vi "Anisotropic Filter Example.vi"() -> ()   [LabVIEW 2012]
uses:
  Non-User VIs/Controls/Anisotropic Filter Parameters.ctl
  User Controls/Array Dimensions.ctl
  <vilib>/Analysis/baseanly.llb/Scale 2D.vi
  Non-User VIs/Allocate Memory/AllocateMemory_32f.vi
  Non-User VIs/Functions/Anisotropic Filter/Create Ansiotropic Filter 32f.vi
  Non-User VIs/Functions/Anisotropic Filter/Compute Anisotropic Filter 32f.vi
  Non-User VIs/Functions/Anisotropic Filter/Delete Ansiotropic Filter 32f.vi
  Non-User VIs/Error Checking/View Error Log Mode Functional Global.vi
  OpenCLV x64.lvlib
  <vilib>/Analysis/NI_AALBase.lvlib
panel:
  in  "Ansiotropic Filter Parameters":T1={"Time Step"=0.1, "Total Time"=0.5, "Std. Deviation"=1.6, "Gaussian Filter X Size"=3, "Gaussian Filter Y Size"=3, "Gaussian Filter Z Size"=3} {"Gaussian Filter Z Size" min=1 max=99 step=2; "Gaussian Filter Y Size" min=1 max=99 step=2; "Gaussian Filter X Size" min=1 max=99 step=2}
  out "Normalized Raw Image":dbl[][](graph)
  out "Normalized Proessed Image":dbl[][](graph)
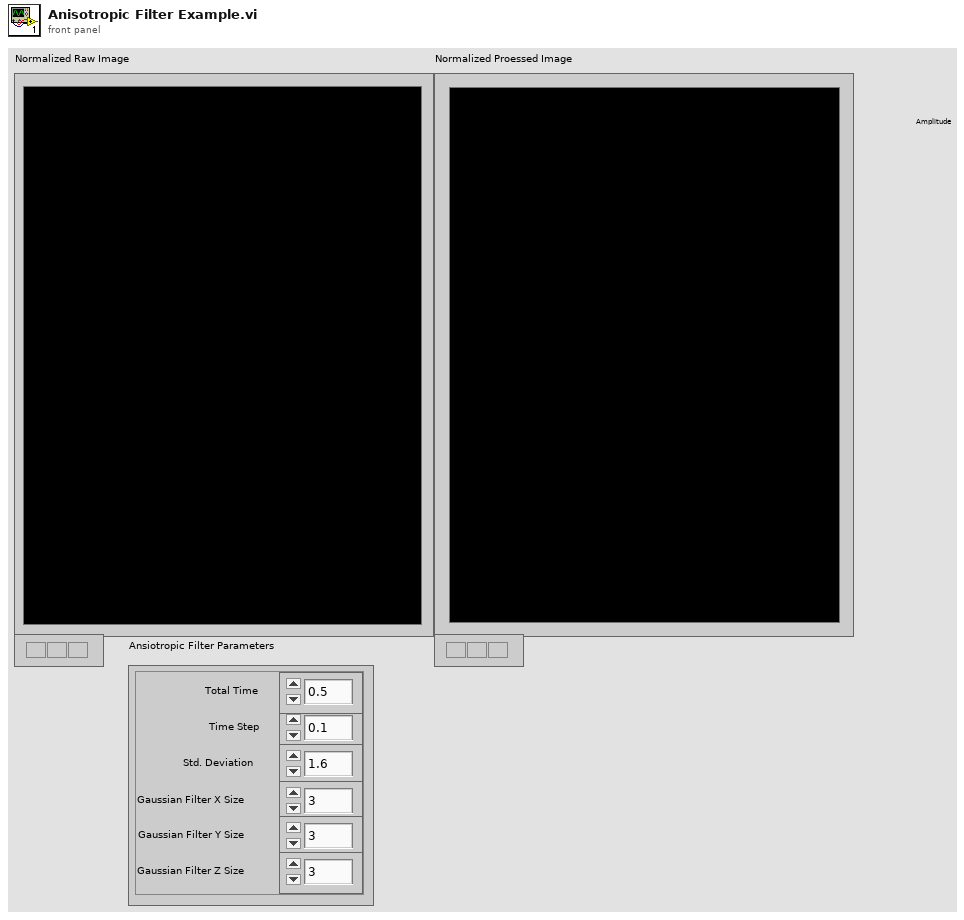
[diagram p1: front panel]
types:
  T1 = typedef "OpenCLV x64.lvlib/Anisotropic Filter Parameters.ctl" = cluster{"Time Step":sgl, "Total Time":sgl, "Std. Deviation":sgl, "Gaussian Filter X Size":u32, "Gaussian Filter Y Size":u32, "Gaussian Filter Z Size":u32}
  T2 = typedef "Array Dimensions.ctl" = cluster{"Depth":u64, "Height":u64, "Width":u64}
  T3 = typedef "imagedata.ctl" = cluster{"image type":i32, "image depth":i32, "image":u8[], "mask":u8[], "colors":u32[], "Rectangle":cluster{"left":i16, "top":i16, "right":i16, "bottom":i16}}
  T4 = typedef "OpenCLV x64.lvlib/Device ID.ctl" = u64
  T5 = typedef "OpenCLV x64.lvlib/Memory Object.ctl" = cluster{"Device ID":T4, "Memeroy ID":T6, "Dimension":T2, "Memory Type":T7}
  T6 = typedef "OpenCLV x64.lvlib/Memory ID.ctl" = u64
  T7 = typedef "OpenCLV x64.lvlib/Memory Type.ctl" = enum16{"32f", "u8", "i8", "u16", "i16", "u32", "i32", "64f"}
  T8 = typedef "OpenCLV x64.lvlib/Anisotropic Filter Object.ctl" = cluster{"Device In":T4, "Convolution Object":T9, "Imag Kernel":sgl[][][], "Real Kernel":sgl[][][], "Convolved Buffer":T5, "Program Handle":T10, "Ansiotropic Filter Parameters":T1, "Raw Data":T5, "Buffer 3":T5, "Dimensions":T2}
  T9 = typedef "OpenCLV x64.lvlib/Convolution Object.ctl" = cluster{"Device In":T4, "Program Handle":T10, "Kernel Memory Object":T5, "Convolved Memory Object":T5}
  T10 = typedef "OpenCLV x64.lvlib/Program Handle.ctl" = u64
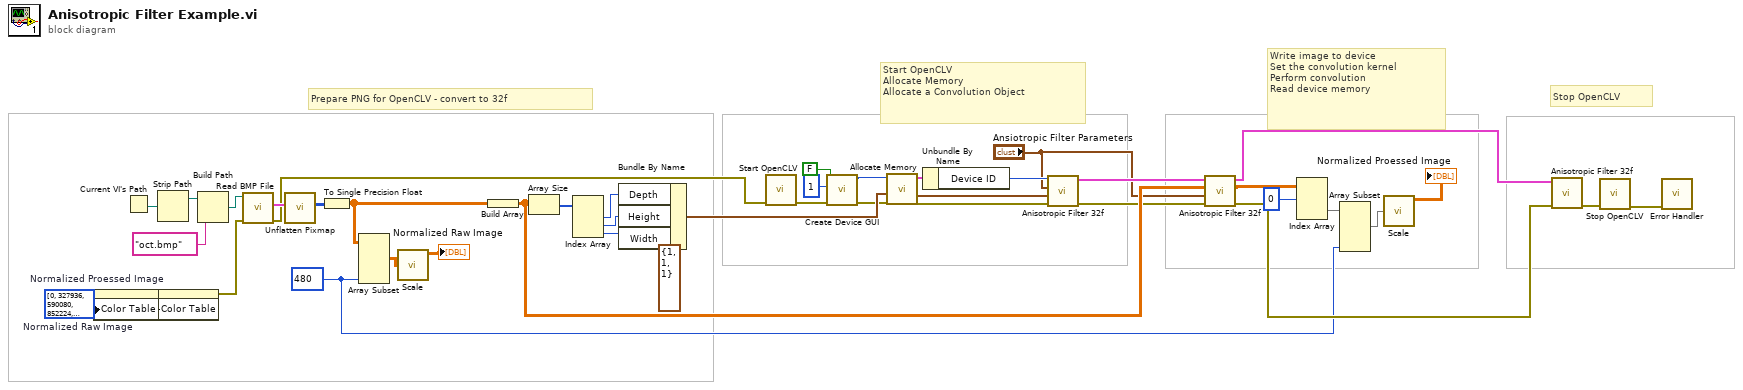
[diagram p0: block diagram]
diagram:
  w1 = 480 ("index")
  w8 = u32[] [0, 327936, 590080, 852224, 983296, 1114624, 1180160, 1311232, 1442304, 1573632, 1704704, 1770240, 1901312, 1966848, 2098176, 2163712, 2294784, 2491392, 2557184, 2688256, 2753792, 2884864, 2950656, 3081728, 3147264, 3344129, 3475457, 3540993, 3672321, 3738113, 3869185, 3934977, 4066305, 4197633, 4328961, 4394497, 4460289, 4591617, 4657409, 4788481, 4854273, 4985601, 5116929, 5248257, 5314049, 5379841, 5511169, 5576961, 5708033, 5773825, 5905153, 6036482, 6167810, 6233346, 6299138, 6430466, 6496258, 6562050, 6693634, 6759426, 6890754, 7022082, 7087874, 7153666, 7284994, 7350786, 7482114, 7547906, 7613698, 7745026, 7876354, 8007682, 8073474, 8139522, 8205314, 8336642, 8467970, 8533763, 8599555, 8665347, 8731139, 8862467, 8993795, 9059587, 9125380, 9191428, 9257220, 9388548, 9454340, 9520132, 9585924, 9717253, 9848837, 9914629, 9980165, 10045957, 10177541, 10243334, 10309126, 10375174, 10440966, 10572294, 10703623, 10769416, 10835208, 10901256, 10967049, 11033097, 11033609, 11099401, 11165450, 11231242, 11231754, 11297547, 11363339, 11429131, 11495180, 11495692, 11561740, 11693069, 11758861, 11759373, 11825165, 11891214, 11957006, 12022799, 12023311, 12089103, 12220944, 12286736, 12286736, 12352529, 12418577, 12484370, 12550162, 12615954, 12681747, 12747796, 12813588, 12813845, 12879894, 12945686, 13077015, 13142808, 13143064, 13208856, 13274905, 13340697, 13340953, 13472282, 13538075, 13604379, 13670172, 13735964, 13801757, 13867550, 13933343, 13999392, 13999648, 14065441, 14131234, 14197027, 14197541, 14263334, 14329383, 14395176, 14460969, 14592553, 14658346, 14724139, 14789932, 14790189, 14856238, 14922287, 14988080, 15053873, 15054130, 15119923, 15185972, 15251765, 15317559, 15383353, 15449146, 15449660, 15515454, 15515968, 15516226, 15582021, 15582278, 15582536, 15648587, 15648844, 15714639, 15714897, 15715155, 15780949, 15781463, 15847256, 15847770, 15848028, 15913823, 15914081, 15979875, 15980133, 15980391, 16046441, 16046444, 16046703, 16046705, 16112500, 16113015, 16113274, 16113277, 16179072, 16179330, 16179588, 16245384, 16245387, 16245389, 16245648, 16311443, 16376982, 16377241, 16377499, 16443294, 16443553, 16443555, 16443815, 16509866, 16510124, 16510127, 16575923, 16575924, 16576182, 16576441, 16576443, 16576702, 16576705, 16576963, 16577222, 16577224, 16577482, 16577485, 16577743, 16577745, 16578004, 16578262, 16578264, 16578523, 16578782, 16579040, 16579299, 16579301, 16579303, 16579562, 16579821] ("Color Table")
  # "Stop OpenCLV"
  # "Write image to device\nSet the convolution kernel\nPerform convolution\nRead device memory"
  # "Start OpenCLV\nAllocate Memory\nAllocate a Convolution Object"
  # "Prepare PNG for OpenCLV - convert to 32f"
  n1 = property on="Normalized Raw Image" class="IntGraph (strict)"("Color Table"=w8) -> (error out=w9:errorcluster)  [unwired: 2 in, 1 out]
  n2 = Current VI's Path() -> (path=w42:path)
  n3 = property on="Normalized Proessed Image" class="IntGraph (strict)"(error in=w9, "Color Table"=w8) -> (error out=w7:errorcluster)  [unwired: 1 in, 1 out]
  n4 = Strip Path(path=w42) -> (stripped path=w41:path)  [unwired: 1 out]
  n5 = Build Path(base path=w41, name or relative path="oct.bmp") -> (appended path=w11:path)
  n6 = call <vilib>:"Read BMP File.vi"("error in (no error)"=w7, "path to BMP file"=w11) -> ("error out"=w10:errorcluster, "image data"=w39:T3)  [unwired: 7 in, 1 out]
  n7 = call <vilib>:"Unflatten Pixmap.vi"("image data"=w39) -> ("8-bit pixmap"=w13:u8[][])  [unwired: 4 in, 6 out]
  n8 = To Single Precision Float(number=w13) -> (single precision float=w5:sgl[][])
  n9 = Array Subset(array=w5, length (col)=w1) -> (w4:sgl[][])  [unwired: 3 in]
  n10 = call-poly <vilib>:"Scale.vi"("X"=w4) -> ("Y=(X-offset)/scale"=→"Normalized Raw Image":dbl[][])  [unwired: 3 out]
  n11 = Build Array(w5) -> (w23:sgl[][][])
  n12 = Array Size(array=w23) -> (size(s)=w35:i32[])
  n13 = Index Array(array=w35) -> (element #1=w31:i32, element #2=w32:i32, element #3=w33:i32)  [unwired: 3 in]
  n14 = Bundle By Name(cluster=T2 {"Depth"=1, "Height"=1, "Width"=1} ("Dimension"), "Depth"=w31, "Height"=w32, "Width"=w33) -> (w29:T2)
  n15 = call "Start OpenCLV.vi"("Error In"=w10) -> ("Error Out"=w38:errorcluster)  [unwired: 10 in]
  n16 = call "Create Device GUI.vi"("Error In"=w38, "Platform"=1, "Skip Configuration"=FALSE) -> ("error constant"=w16:errorcluster, "Device Reference"=w17:T4)  [unwired: 7 in]
  n17 = call-poly "Allocate Memory.vi"("Error In"=w16, "Dimension"=w29, "Device In"=w17) -> ("Error Out"=w27:errorcluster, "Dimension Out"=w25:T2, "Memory Object"=w28:T5)  [unwired: 6 in]
  n18 = Unbundle By Name(w28) -> ("Device ID"=w26:T4)
  n19 = call-poly "Anisotropic Filter 32f.vi"("Error In"=w27, "Dimensions"=w25, "Ansiotropic Filter Parameters"="Ansiotropic Filter Parameters", "Device In"=w26) -> ("Error Out"=w22:errorcluster, "Anisotropic Filter Object"=w24:T8)  [unwired: 6 in]
  n20 = call-poly "Anisotropic Filter 32f.vi"("Error In"=w22, "Anisotropic Filter Parameters"="Ansiotropic Filter Parameters", "Data In"=w23, "Anisotropic Filter Object"=w24) -> ("Error Out"=w18:errorcluster, "Data Out"=w21:sgl[][][], "Anisotropic Filter Object Out"=w19:T8)  [unwired: 4 in, 1 out]
  n21 = Index Array(array=w21, index (dim 0)=0 ("index (page)")) -> (element=w3:sgl[][])  [unwired: 2 in]
  n22 = Array Subset(array=w3, length (col)=w1) -> (w2:sgl[][])  [unwired: 3 in]
  n23 = call-poly <vilib>:"Scale.vi"("X"=w2) -> ("Y=(X-offset)/scale"=→"Normalized Proessed Image":dbl[][])  [unwired: 3 out]
  n24 = call-poly "Anisotropic Filter 32f.vi"("Error In"=w18, "Anisotropic Filter Object"=w19) -> ("Error Out"=w20:errorcluster)  [unwired: 9 in]
  n25 = call "Stop OpenCLV.vi"("Error In"=w20) -> ("Error Out"=w6:errorcluster)  [unwired: 10 in]
  n26 = call-poly "Error Handler.vi"("Error In"=w6) -> ()  [unwired: 10 in, 1 out]
